vi "Launch Watch Loop.vi"(8 "error in (no error)":errorcluster, 11 "WebProjectWatcher in":refnum<class "WebProjectWatcher.lvclass">) -> (0 "error out":errorcluster, 3 "WebProjectWatcher out":refnum<class "WebProjectWatcher.lvclass">)   [LabVIEW 2020, in "PicoG-Processor.lvlib" / "WebProjectWatcher.lvclass"]
uses:
  WebProjectWatcher.lvclass
  Watch Loop Async.vi
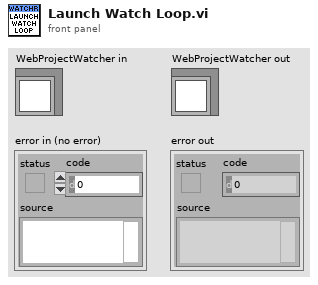
[diagram p1: front panel]
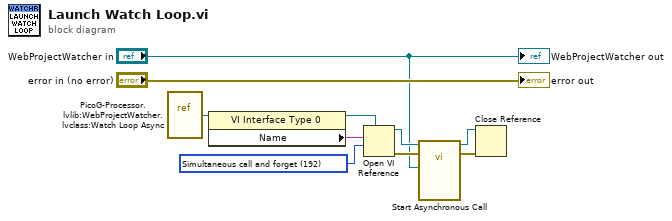
[diagram p0: block diagram]
diagram:
  w4 = 192 items=["Record modifications"=1, "Open templates for editing"=2, "Prompt user to save"=4, "Prepare for reentrant run"=8, "Prompt to find missing subVIs"=16, "Hide loading dialog box"=32, "Enable simultaneous calls"=64, "Prepare to call and forget"=128, "Simultaneous call and forget"=192, "Prepare to call and collect"=256, "Simultaneous call and collect"=320]
  n1 = vi-ref "PicoG-Processor.lvlib:WebProjectWatcher.lvclass:Watch Loop Async.vi"() -> (w2:refnum<vi>)
  n2 = property class="VI Interface Type 0"(reference=w2) -> (reference out=w5:refnum<vi>, "Name"=w3:string)  [unwired: 1 in, 1 out]
  n3 = Open VI Reference(type specifier VI Refnum (for type only)=w5, vi path=w3, options=w4) -> (vi reference=w7:refnum<vi>, error out=w6:errorcluster)  [unwired: 3 in]
  n4 = call-by-ref "Start Asynchronous Call"(reference=w7, error in=w6, "WebProjectWatcher in"="WebProjectWatcher in") -> (reference out=w9:refnum<vi>, error out=w8:errorcluster)  [unwired: 11 in]
  n5 = Close Reference(reference=w9, error in (no error)=w8) -> ()  [unwired: 1 out]
  "error out" <- "error in (no error)"
  "WebProjectWatcher out" <- "WebProjectWatcher in"
